vi "SysDef.Version.Get.vi"(8 "error in (no error)":errorcluster, 11 "nodeID":u64) -> (0 "error out":errorcluster, 2 "Version":string, 3 "nodeID out":u64)   [LabVIEW 2027, in "Advanced System Definition.lvlib"]
uses:
  Advanced System Definition.lvlib
  C:/NetCore/niveristand-custom-device-development-tools/advanced-sysdef-api/Source/SysDef API/SysDef.Version.Get.vi/NationalInstruments.VeriStand.SystemDefinitionAPI
  NationalInstruments.VeriStand.SystemDefinitionAPI
  <vilib>/NI VeriStand/Custom Device API/Custom Device API.lvlib
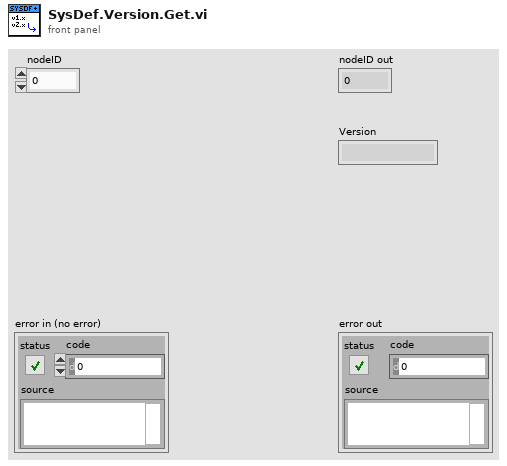
[diagram p1: front panel]
types:
  T1 = typedef "Custom Device API.lvlib/Custom Device Item Ref.ctl" = u64
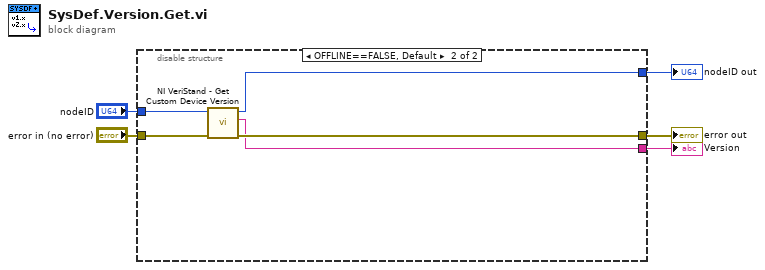
[diagram p0: block diagram]
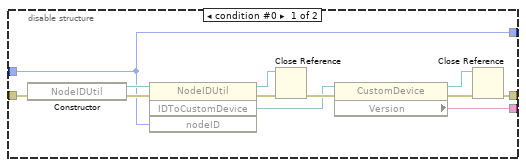
[diagram p2: hidden frame]
diagram:
  n1 = disable-structure shown="OFFLINE==FALSE, Default" {
    disable-tunnel: "error in (no error)" -> [w12 w21]
    disable-tunnel: "nodeID" -> [w9 w22]
    disable-tunnel: [w6 w20] -> w3
    disable-tunnel: [w7 w18] -> w2
    disable-tunnel: [w9 w19] -> w1
    frame condition #0 {
      n2 = constructor class="NodeIDUtil"(error in=w12) -> (reference out=w17:refnum<k24>, error out=w16:errorcluster)  [unwired: 2 in, 1 out]
      n3 = invoke class="NodeIDUtil" method="IDToCustomDevice"(reference=w17, error in=w16, "nodeID"=w9) -> (reference out=w13:refnum<k24>, error out=w15:errorcluster, "IDToCustomDevice"=w8:refnum<k24>)  [unwired: 1 in, 1 out]
      n4 = Close Reference(reference=w13, error in (no error)=w15) -> (error out=w14:errorcluster)
      n5 = property class="CustomDevice"(reference=w8, error in=w14) -> (reference out=w11:refnum<k24>, error out=w10:errorcluster, "Version"=w7:string)
      n6 = Close Reference(reference=w11, error in (no error)=w10) -> (error out=w6:errorcluster)
    }
    frame condition #1 (active) {
      n7 = call <vilib>:"NI VeriStand - Get Custom Device Version.vi"("error in (no error)"=w21, "Device Ref in"=w22) -> ("error out"=w20:errorcluster, "Value"=w18:string, "Device Ref out"=w19:T1)  [unwired: 7 in]
    }
  }
  "nodeID out" <- w1
  "error out" <- w3
  "Version" <- w2
